vi "RecordPath.vi"(8 "error in":errorcluster caption="错误输入", 11 "Path":string="Config\\data.ini") -> (0 "error out":errorcluster caption="错误输出", 3 "PathOut":path)   [LabVIEW 2013]
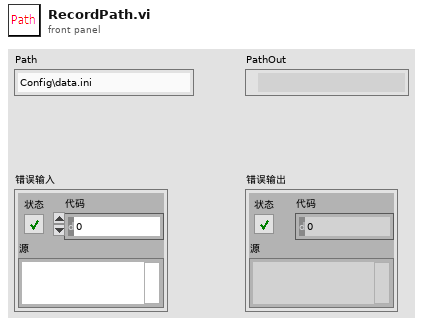
[diagram p1: front panel]
types:
  T1 = enum32{"invalid app kind", "Development System", "Run Time System", "Student Edition", "Embedded LabVIEW", "Evaluation", "Custom"}
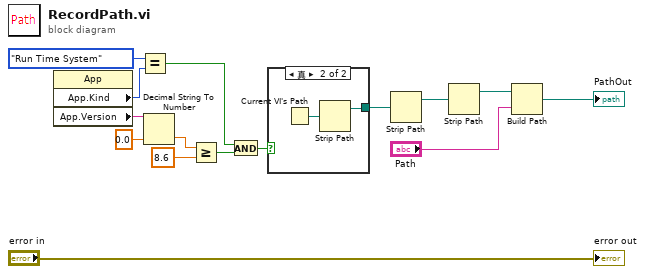
[diagram p0: block diagram]
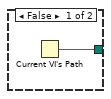
[diagram p2: hidden frame]
diagram:
  n1 = property class="App"() -> ("App.Kind"=w11:T1, "App.Version"=w12:string)  [unwired: 2 in, 2 out]
  n2 = Equal?(x=T1."Run Time System", y=w11) -> (x = y?=w8:bool)
  n3 = Decimal String To Number(string=w12, default (0L)=0.0 ("y")) -> (number=w14:dbl)  [unwired: 1 in, 1 out]
  n4 = Greater Or Equal?(x=w14, y=8.6) -> (x >= y?=w7:bool)
  n5 = And(x=w8, y=w7) -> (x .and. y?=w9:bool)
  n6 = case shown="真" w9 {
    tunnel: [w16 w17] -> w4
    frame False {
      n7 = Current VI's Path() -> (path=w16:path)
    }
    frame True {
      n8 = Current VI's Path() -> (path=w18:path)
      n9 = Strip Path(path=w18) -> (stripped path=w17:path)  [unwired: 1 out]
    }
  }
  n10 = Strip Path(path=w4) -> (stripped path=w3:path)  [unwired: 1 out]
  n11 = Strip Path(path=w3) -> (stripped path=w6:path)  [unwired: 1 out]
  n12 = Build Path(base path=w6, name or relative path="Path") -> (appended path=→"PathOut":path)
  "error out" <- "error in"
